vi "EtherNet CIP WriteBit_Array.vi"(0 "Connection Cluster":T1={"TCP Connection"=refnum, "Session"=[], "EtherNet/IP Device Address"="172.20.37.243"} {"Session" format="0x%02x"}, 5 "Tag":string, 9 "BOOL Array":bool[](array[boolean]), 11 "error in":errorcluster) -> (4 "Connection Cluster Out":T1, 15 "error out":errorcluster)   [LabVIEW 2012]
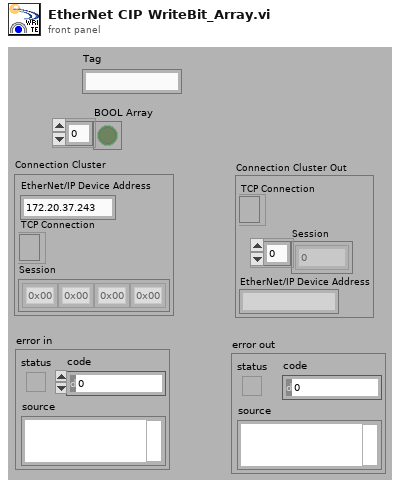
[diagram p1: front panel]
types:
  T1 = cluster{"TCP Connection":refnum<k5>, "Session":u8[], "EtherNet/IP Device Address":string}
  T2 = enum16{"No Data", "BOOL", "BIT Array", "SINT", "INT", "DINT", "REAL", "TIMER/CONTROL/COUNTER"}
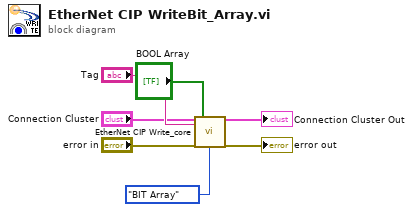
[diagram p0: block diagram]
diagram:
  n1 = call "EtherNet CIP Write_core.vi"("Connection Cluster"="Connection Cluster", "Tag"="Tag", "error in"="error in", "BOOL Array"="BOOL Array", "Datatype"=T2."BIT Array") -> ("Connection Cluster Out"=→"Connection Cluster Out":T1, "error out"=→"error out":errorcluster)  [unwired: 13 in]
